vi "PH_Cam_BaseClass.draw Center Cross.vi"(0 "Image In":T1, 1 "X Resolution":i32, 2 "Y Resolution":i32, 3 "Scale Factor":dbl, 5 "error in (no error)":errorcluster, 9 "Color":u32(colorbox)=3381759) -> (14 "Image Out":T1, 19 "error out":errorcluster)   [LabVIEW 2014, in "PH_Cam_BaseClass.lvlib"]
doc: "This VI overlays a center cross to the image."
uses:
  <vilib>/vision/Image Controls.llb/IMAQ Image.ctl
  PH_Cam_BaseClass.lvlib
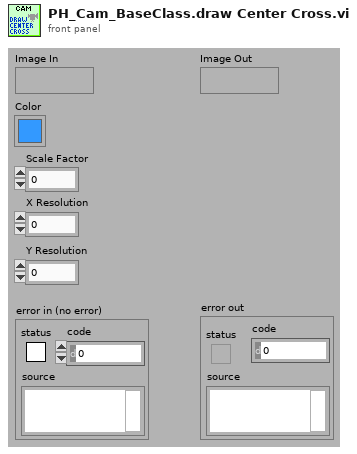
[diagram p1: front panel]
types:
  T1 = typedef "IMAQ Image.ctl" = refnum<image>
  T2 = cluster{"Left":i32, "Top":i32, "Right":i32, "Bottom":i32}
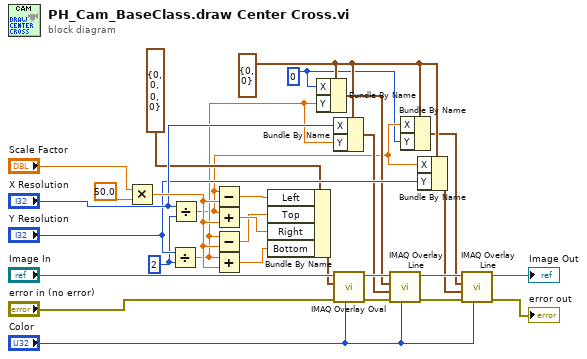
[diagram p0: block diagram]
diagram:
  w1 = 0 ("X")
  w6 = cluster{"X":i32, "Y":i32} {"X"=0, "Y"=0} ("Start Point")
  w17 = 2 ("y")
  n1 = Multiply(x="Scale Factor", y=50.0) -> (x*y=w29:dbl)
  n2 = Divide(x="Y Resolution", y=w17) -> (x/y=w3:dbl)
  n3 = Divide(x="X Resolution", y=w17) -> (x/y=w2:dbl)
  n4 = Subtract(x=w2, y=w29) -> (x-y=w16:dbl)
  n5 = Add(x=w2, y=w29) -> (x+y=w15:dbl)
  n6 = Subtract(x=w3, y=w29) -> (x-y=w14:dbl)
  n7 = Add(x=w3, y=w29) -> (x+y=w13:dbl)
  n8 = Bundle By Name(cluster=T2 {"Left"=0, "Top"=0, "Right"=0, "Bottom"=0} ("Bounding Rectangle"), "Left"=w16, "Top"=w14, "Right"=w15, "Bottom"=w13) -> (w18:T2)
  n9 = Bundle By Name(cluster=w6, "X"=w1, "Y"=w3) -> (w7:cluster{"X":i32, "Y":i32})
  n10 = Bundle By Name(cluster=w6, "X"="X Resolution", "Y"=w3) -> (w8:cluster{"X":i32, "Y":i32})
  n11 = call "IMAQ Overlay Oval"("Color"="Color", "error in (no error)"="error in (no error)", "Bounding Rectangle"=w18, "Image"="Image In") -> ("error out"=w11:errorcluster, "Image Out"=w9:T1)  [unwired: 6 in]
  n12 = call "IMAQ Overlay Line"("Color"="Color", "error in (no error)"=w11, "End Point"=w8, "Start Point"=w7, "Image"=w9) -> ("error out"=w12:errorcluster, "Image Out"=w10:T1)  [unwired: 5 in]
  n13 = Bundle By Name(cluster=w6, "X"=w2, "Y"=w1) -> (w5:cluster{"X":i32, "Y":i32})
  n14 = Bundle By Name(cluster=w6, "X"=w2, "Y"="Y Resolution") -> (w4:cluster{"X":i32, "Y":i32})
  n15 = call "IMAQ Overlay Line"("Color"="Color", "error in (no error)"=w12, "End Point"=w4, "Start Point"=w5, "Image"=w10) -> ("error out"=→"error out":errorcluster, "Image Out"=→"Image Out":T1)  [unwired: 5 in]
